vi "Chart_Create evenly-spaced dataset.vi"(6 "Initialize?":bool, 9 "X-Axis Time Interval (100) [ms]":i32, 10 "X (Time Stamp)":timestamp, 11 "Y (DBL)":dbl) -> (2 "X (Interpolated array)":timestamp[](array[timestamp]), 3 "Y (Interpolated array)":dbl[](array[numeric]))   [LabVIEW 2019]
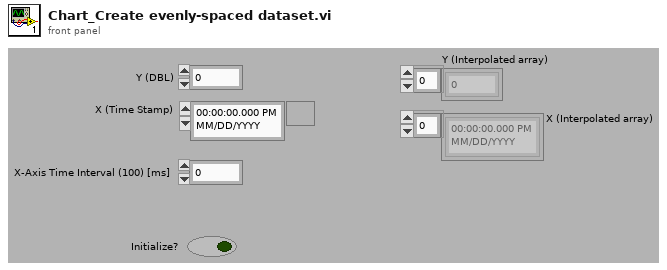
[diagram p1: front panel]
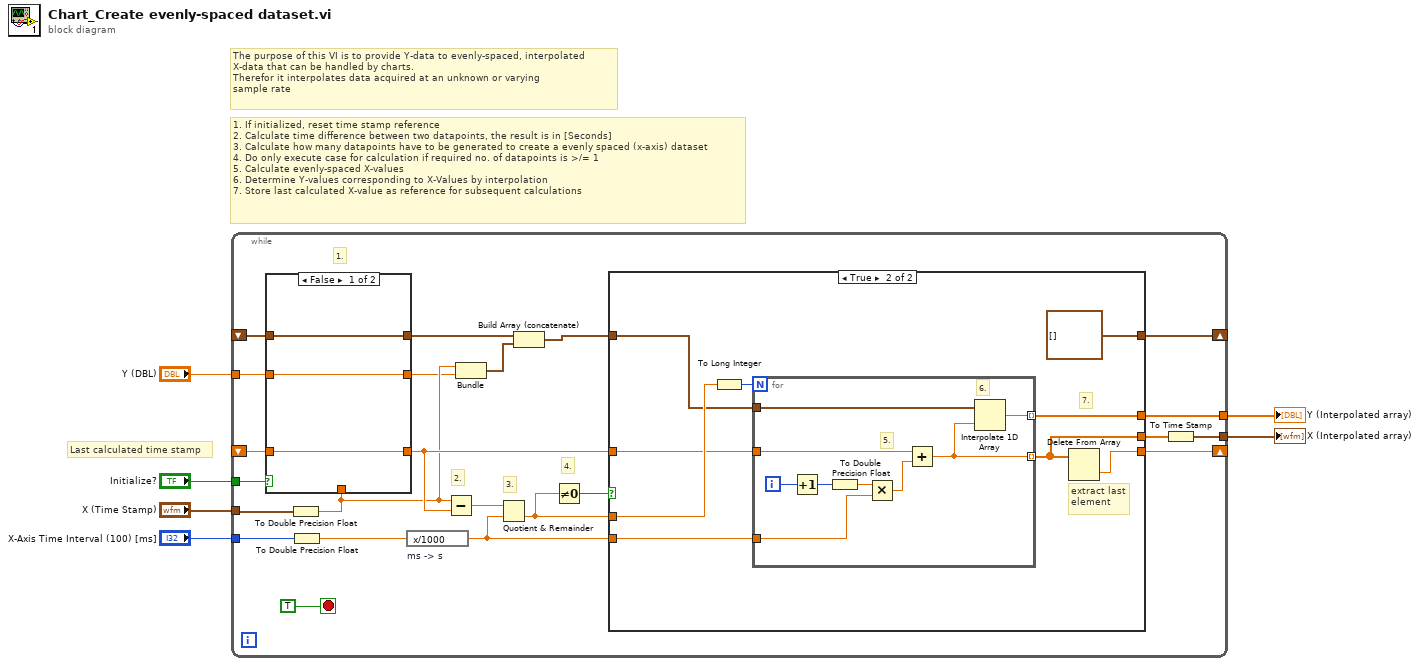
[diagram p0: block diagram]
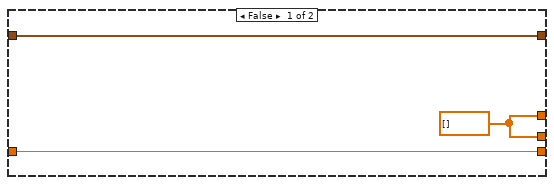
[diagram p2: hidden frame]
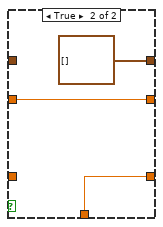
[diagram p3: hidden frame]
diagram:
  # "The purpose of this VI is to provide Y-data to evenly-spaced, interpolated\nX-data that can be handled by charts.\nTherefor it interpolates data acquired at an unknown or varying\nsample rate"
  # "Last calculated time stamp"
  # "1. If initialized, reset time stamp reference\n2. Calculate time difference between two datapoints, the result is in [Seconds]\n3. Calculate how many datapoints have to be generated to create a evenly spaced (x-axis) dataset\n4. Do only execute case for calculation if required no. of datapoints is >/= 1\n5. Calculate evenly-spaced X-values\n6. Determine Y-values corresponding to X-Values by interpolation \n7. Store last calculated X-value as reference for subsequent calculations"
  n1 = while {
    tunnel: "Y (DBL)" -> [w15]
    tunnel: "X-Axis Time Interval (100) [ms]" -> [w24]
    tunnel: "X (Time Stamp)" -> [w18]
    shift-right: [w26] -> _
    shift-left: _ -> [w28]
    tunnel: "Initialize?" -> [w29]
    tunnel: [w14] -> w2
    tunnel: [w12] -> w1
    shift-right: [w9] -> _
    shift-left: _ -> [w7]
    stop <- TRUE ("stop") stop-if-true
    # "4."
    # "3."
    # "2."
    # "1."
    n2 = To Double Precision Float(number=w18) -> (double precision float=w17:dbl)
    n3 = case shown="False" w29 {
      tunnel: w17 -> [_ w56]
      tunnel: w28 -> [w53 _]
      tunnel: [w53 w56] -> w25
      tunnel: [w52 w55] -> w16
      tunnel: w15 -> [w52 w55]
      tunnel: [w51 cluster{dbl, "Y (DBL)":dbl}[] []] -> w8
      tunnel: w7 -> [w51 _]
      frame False {
      }
      frame True {
      }
    }
    n4 = To Double Precision Float(number=w24) -> (double precision float=w21:dbl)
    n5 = expression code="x/1000" "ms -> s"(w21) -> (w22:dbl)
    n6 = Subtract(x=w17, y=w25) -> (x-y=w23:dbl)
    n7 = Bundle(w17, "Y (DBL)"=w16) -> (w10:cluster{dbl, "Y (DBL)":dbl})  [unwired: 1 in]
    n8 = Quotient & Remainder(x=w23, y=w22) -> (floor(x/y)=w19:dbl)  [unwired: 1 out]
    n9 = Build Array (concatenate)(w8, w10) -> (w11:cluster{dbl, "Y (DBL)":dbl}[])
    n10 = Not Equal To 0?(x=w19) -> (x != 0?=w20:bool)
    n11 = case shown="True" w20 {
      tunnel: w25 -> [w32 w37]
      tunnel: [w32 w38] -> w26
      tunnel: w19 -> [_ w40]
      tunnel: w22 -> [_ w39]
      tunnel: [w30 w36] -> w14
      tunnel: [w30 w35] -> w13
      tunnel: w11 -> [w31 w34]
      tunnel: [w31 cluster{dbl, "Y (DBL)":dbl}[] []] -> w9
      frame False {
        w30 = dbl[] []
      }
      frame True {
        # "7."
        # "extract last\nelement"
        n12 = To Long Integer(number=w40) -> (32bit integer=w41:i32)
        n13 = for {
          N: w41 -> [_]
          tunnel: w37 -> [w50]
          tunnel: w39 -> [w47]
          tunnel: [w44] -> w35 mode=indexing
          tunnel: w34 -> [w43]
          tunnel: [w42] -> w36 mode=indexing
          i -> [w49]
          # "6."
          # "5."
          n14 = Increment(x=w49) -> (x+1=w48:i32)
          n15 = To Double Precision Float(number=w48) -> (double precision float=w46:dbl)
          n16 = Multiply(x=w46, y=w47) -> (x*y=w45:dbl)
          n17 = Add(x=w50, y=w45) -> (x+y=w44:dbl)
          n18 = Interpolate 1D Array(1:w44, 2:w43) -> (0:w42:dbl)
        }
        n19 = Delete From Array(array=w35) -> (deleted portion=w38:dbl)  [unwired: 2 in, 1 out]
      }
    }
    n20 = To Time Stamp(1:w13) -> (0:w12:timestamp[])
  }
  "Y (Interpolated array)" <- w2
  "X (Interpolated array)" <- w1
